vi "DetectDev.vi"(1 "IP.":string caption="IP地址") -> (0 "Fail":bool)   [LabVIEW 2012]
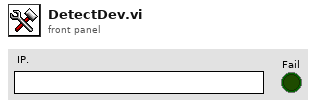
[diagram p1: front panel]
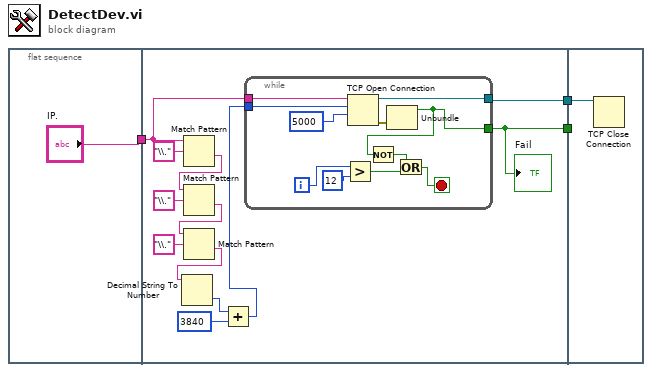
[diagram p0: block diagram]
diagram:
  n1 = flat-sequence {
    tunnel: ["IP."] -> w3
    tunnel: w3 -> [w11]
    tunnel: [w6] -> w2
    tunnel: [w5] -> w1
    tunnel: w2 -> [w28]
    tunnel: w1 -> [_]
    frame #0 {
    }
    frame #1 {
      n2 = Match Pattern(string=w11, regular expression="\\." ("正则表达式")) -> (after substring=w13:string)  [unwired: 1 in, 3 out]
      n3 = Match Pattern(string=w13, regular expression="\\." ("正则表达式")) -> (after substring=w12:string)  [unwired: 1 in, 3 out]
      n4 = Match Pattern(string=w12, regular expression="\\." ("正则表达式")) -> (after substring=w10:string)  [unwired: 1 in, 3 out]
      n5 = Decimal String To Number(string=w10) -> (number=w9:i32)  [unwired: 2 in, 1 out]
      n6 = Add(x=w9, y=3840) -> (x+y=w7:i32)
      n7 = while {
        tunnel: w11 -> [w27]
        tunnel: w7 -> [w26]
        tunnel: [w25] -> w6
        tunnel: [w17] -> w5
        i -> [w22]
        stop <- w19 stop-if-true
        n8 = Greater?(x=w22, y=12) -> (0:w20:bool)
        n9 = TCP Open Connection(address=w27, remote port or service name=w26, timeout ms (60000)=5000 ("超时毫秒(60000)")) -> (connection ID=w25:refnum<k5>, error out=w23:errorcluster)  [unwired: 2 in]
        n10 = Unbundle(w23) -> ("status"=w17:bool)  [unwired: 2 out]
        n11 = Not(x=w17) -> (.not. x?=w18:bool)
        n12 = Or(x=w18, y=w20) -> (x .or. y?=w19:bool)
      }
      "Fail" <- w5
    }
    frame #2 {
      n13 = TCP Close Connection(connection ID=w28) -> ()  [unwired: 2 in, 2 out]
    }
  }
